vi "Fixturing Subtraction Point Tool Histogram.vi"(9 "ROI IN":T1, 10 "Fixturing ROI":i32[](array[numeric])=[0, 0, 0, 0]) -> (2 "ROI OUT":T1, 3 "Rectangle out":i32[](array[numeric]))   [LabVIEW 2020]
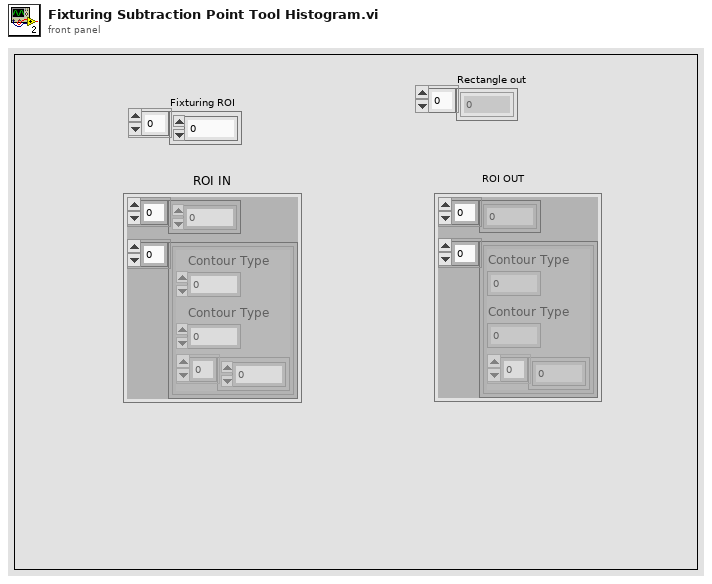
[diagram p1: front panel]
types:
  T1 = cluster{i32[], cluster{"Contour Type":u32, "Contour Type":i32, i32[]}[]}
  T2 = cluster{"Contour Type":u32, "Contour Type":i32, i32[]}[]
  T3 = cluster{"Contour Type":u32, "Contour Type":i32, i32[]}
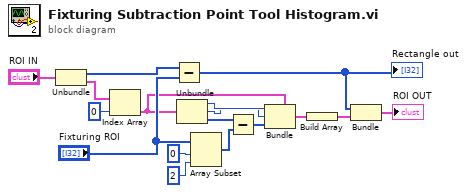
[diagram p0: block diagram]
diagram:
  n1 = Unbundle("ROI IN") -> (w14:i32[], w12:T2)
  n2 = Index Array(array=w12, index=0) -> (element=w9:T3)
  n3 = Subtract(x=w14, y="Fixturing ROI") -> (x-y=w5:i32[])
  "Rectangle out" <- w5
  n4 = Unbundle(w9) -> ("Contour Type"=w3:u32, "Contour Type"=w2:i32, w11:i32[])
  n5 = Array Subset(array="Fixturing ROI", index=0, length=2) -> (w10:i32[])
  n6 = Subtract(x=w11, y=w10) -> (x-y=w8:i32[])
  n7 = Bundle(cluster=w9, "Contour Type"=w3, "Contour Type"=w2, w8) -> (w7:T3)
  n8 = Build Array(w7) -> (w6:T2)
  n9 = Bundle(w5, w6) -> (→"ROI OUT":T1)  [unwired: 1 in]
